vi "HypervisorWrite.vi"(8 "ErrorIn":errorcluster, 10 "EventToLog":T1, 11 "QIn":refnum<queue>) -> (0 "ErrorOut":errorcluster, 3 "QOut":refnum<queue>)   [LabVIEW 2018]
doc: "This VI writes EventToLog to the Hypervisor log file.\n\nCopyright © 2011 Epimedia, Inc. All Rights Reserved.\n\nThe Epimedia Application Library is Copyright © 2009-2011 Epimedia, Inc. \nAll Rights Reserved. Used under license."
uses:
  HyperVisor.ctl
panel:
  # "Copyright © 2011 Epimedia, Inc. All Rights Reserved.\n\nThe Epimedia Application Library is Copyright © 2009-2011 Epimedia, Inc. \nAll Rights Reserved. Used under license."
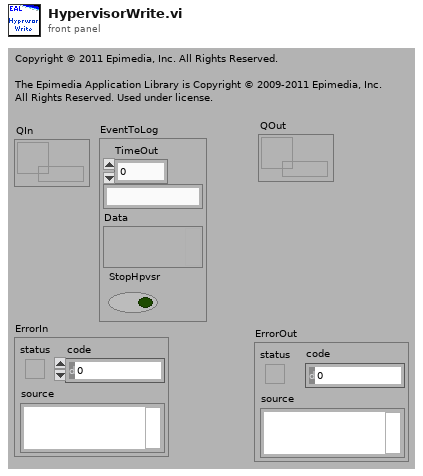
[diagram p1: front panel]
types:
  T1 = typedef "HyperVisor.ctl" = cluster{"TimeOut":dbl, string, "Data":variant, "StopHpvsr":bool}
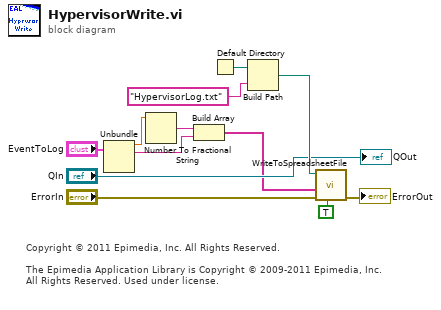
[diagram p0: block diagram]
diagram:
  # "Copyright © 2011 Epimedia, Inc. All Rights Reserved.\n\nThe Epimedia Application Library is Copyright © 2009-2011 Epimedia, Inc. \nAll Rights Reserved. Used under license."
  n1 = Unbundle("EventToLog") -> ("TimeOut"=w9:dbl, w8:string)  [unwired: 2 out]
  n2 = Number To Fractional String(number=w9) -> (F-format string=w7:string)  [unwired: 1 in, 2 out]
  n3 = Build Array(w7, w8) -> (w3:string[])
  n4 = Default Directory() -> (w1:path)
  n5 = Build Path(base path=w1, name or relative path="HypervisorLog.txt") -> (appended path=w10:path)
  n6 = call "WriteToSpreadsheetFile.vi"("Append?(NewFile:F)"=TRUE ("append to file? (new file:F)"), "ErrorIn"="ErrorIn", "1D-Data"=w3, "FilePath(DialogIfEmpty)"=w10) -> ("ErrorOut"=→"ErrorOut":errorcluster)  [unwired: 4 in, 3 out]
  "QOut" <- "QIn"
